vi "setSerializedData.vi"(0 "reference":refnum<class "PackageNode.lvclass">, 1 "parent":refnum<class "AbstractNode.lvclass">, 2 "children":refnum<class "AbstractNode.lvclass">[](array[class]), 3 "xmlOut":string, 5 "error in (no error)":errorcluster) -> (14 "reference out":refnum<class "PackageNode.lvclass">, 19 "error out":errorcluster)   [LabVIEW 2014, in "PackageNode.lvclass"]
doc: "setSerializedData"
uses:
  <resource>/Framework/Providers/Open_GDS/UML/PackageNode_class/PackageNode.lvclass
  <resource>/Framework/Providers/Open_GDS/UML/AbstractNode_class/AbstractNode.lvclass
  <resource>/Framework/Providers/Open_GDS/UML/General/Rectangle/Rectangle Rectangle2D.ctl
  <resource>/Framework/Providers/Open_GDS/UML/MultiLineString_class/JustificationType.ctl
  <resource>/Framework/Providers/Open_GDS/UML/MultiLineString_class/MultiLineString.lvclass
  <resource>/Framework/Providers/Open_GDS/UML/RectangularNode_class/RectangularNode.lvclass
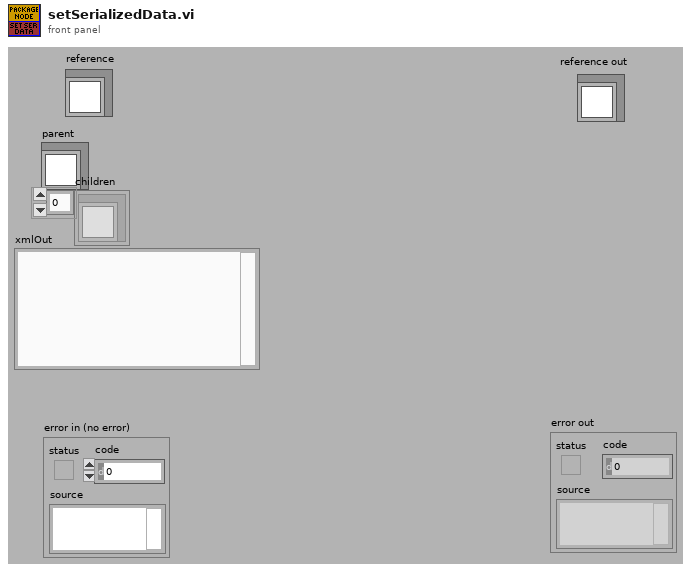
[diagram p1: front panel]
types:
  T1 = typedef "Rectangle Rectangle2D.ctl" = cluster{"x":dbl, "y":dbl, "width":dbl, "height":dbl}
  T2 = cluster{"Base class":cluster{"Base class":cluster{"parent":refnum<k1>, "children":refnum<k1>[], "Hidden":bool}, "bounds":T1}, "name":string, "contents":refnum<k1>, "DEFAULT_TOP_WIDTH":i32, "DEFAULT_TOP_HEIGHT":i32, "DEFAULT_WIDTH":i32, "DEFAULT_HEIGHT":i32, "NAME_GAP":i32, "XGAP":i32, "YGAP":i32, "Collapsed":bool, "Note color":u32, "Justification":u16}
  T3 = cluster{"Base class":cluster{"Base class":cluster{"parent":refnum<k1>, "children":refnum<k1>[], "Hidden":bool}, "bounds":T1}, "name":string, "contents":refnum<k1>, "DEFAULT_TOP_WIDTH":i32, "DEFAULT_TOP_HEIGHT":i32, "DEFAULT_WIDTH":i32, "DEFAULT_HEIGHT":i32, "NAME_GAP":i32, "XGAP":i32, "YGAP":i32, "Collapsed":bool}
  T4 = typedef "MultiLineString.lvclass/JustificationType.ctl" = enum16{"LEFT", "CENTER", "RIGHT"}
  T5 = cluster{"Attributes":cluster{"Base class":cluster{"Base class":cluster{"parent":refnum<k1>, "children":refnum<k1>[], "Hidden":bool}, "bounds":T1}, "name":string, "contents":refnum<k1>, "DEFAULT_TOP_WIDTH":i32, "DEFAULT_TOP_HEIGHT":i32, "DEFAULT_WIDTH":i32, "DEFAULT_HEIGHT":i32, "NAME_GAP":i32, "XGAP":i32, "YGAP":i32, "Collapsed":bool, "Note color":u32, "Justification":u16}, string}
  T6 = typedef "RectangularNode.lvclass/ObjectAttributes.ctl" = cluster{"bounds":T1}
  T7 = typedef "AbstractNode.lvclass/ObjectAttributes.ctl" = cluster{"parent":refnum<class "AbstractNode.lvclass">, "children":refnum<class "AbstractNode.lvclass">[], "Hidden":bool}
  T8 = typedef "PackageNode.lvclass/ObjectAttributes.ctl" = cluster{"name":string, "contents":refnum<class "MultiLineString.lvclass">, "DEFAULT_TOP_WIDTH":i32, "DEFAULT_TOP_HEIGHT":i32, "DEFAULT_WIDTH":i32, "DEFAULT_HEIGHT":i32, "NAME_GAP":i32, "XGAP":i32, "YGAP":i32, "Collapsed":bool, "Note color":u32, "Justification":u16}
  T9 = cluster{"Attributes":cluster{"Base class":cluster{"Base class":cluster{"parent":refnum<k1>, "children":refnum<k1>[], "Hidden":bool}, "bounds":T1}, "name":string, "contents":refnum<k1>, "DEFAULT_TOP_WIDTH":i32, "DEFAULT_TOP_HEIGHT":i32, "DEFAULT_WIDTH":i32, "DEFAULT_HEIGHT":i32, "NAME_GAP":i32, "XGAP":i32, "YGAP":i32, "Collapsed":bool}, string}
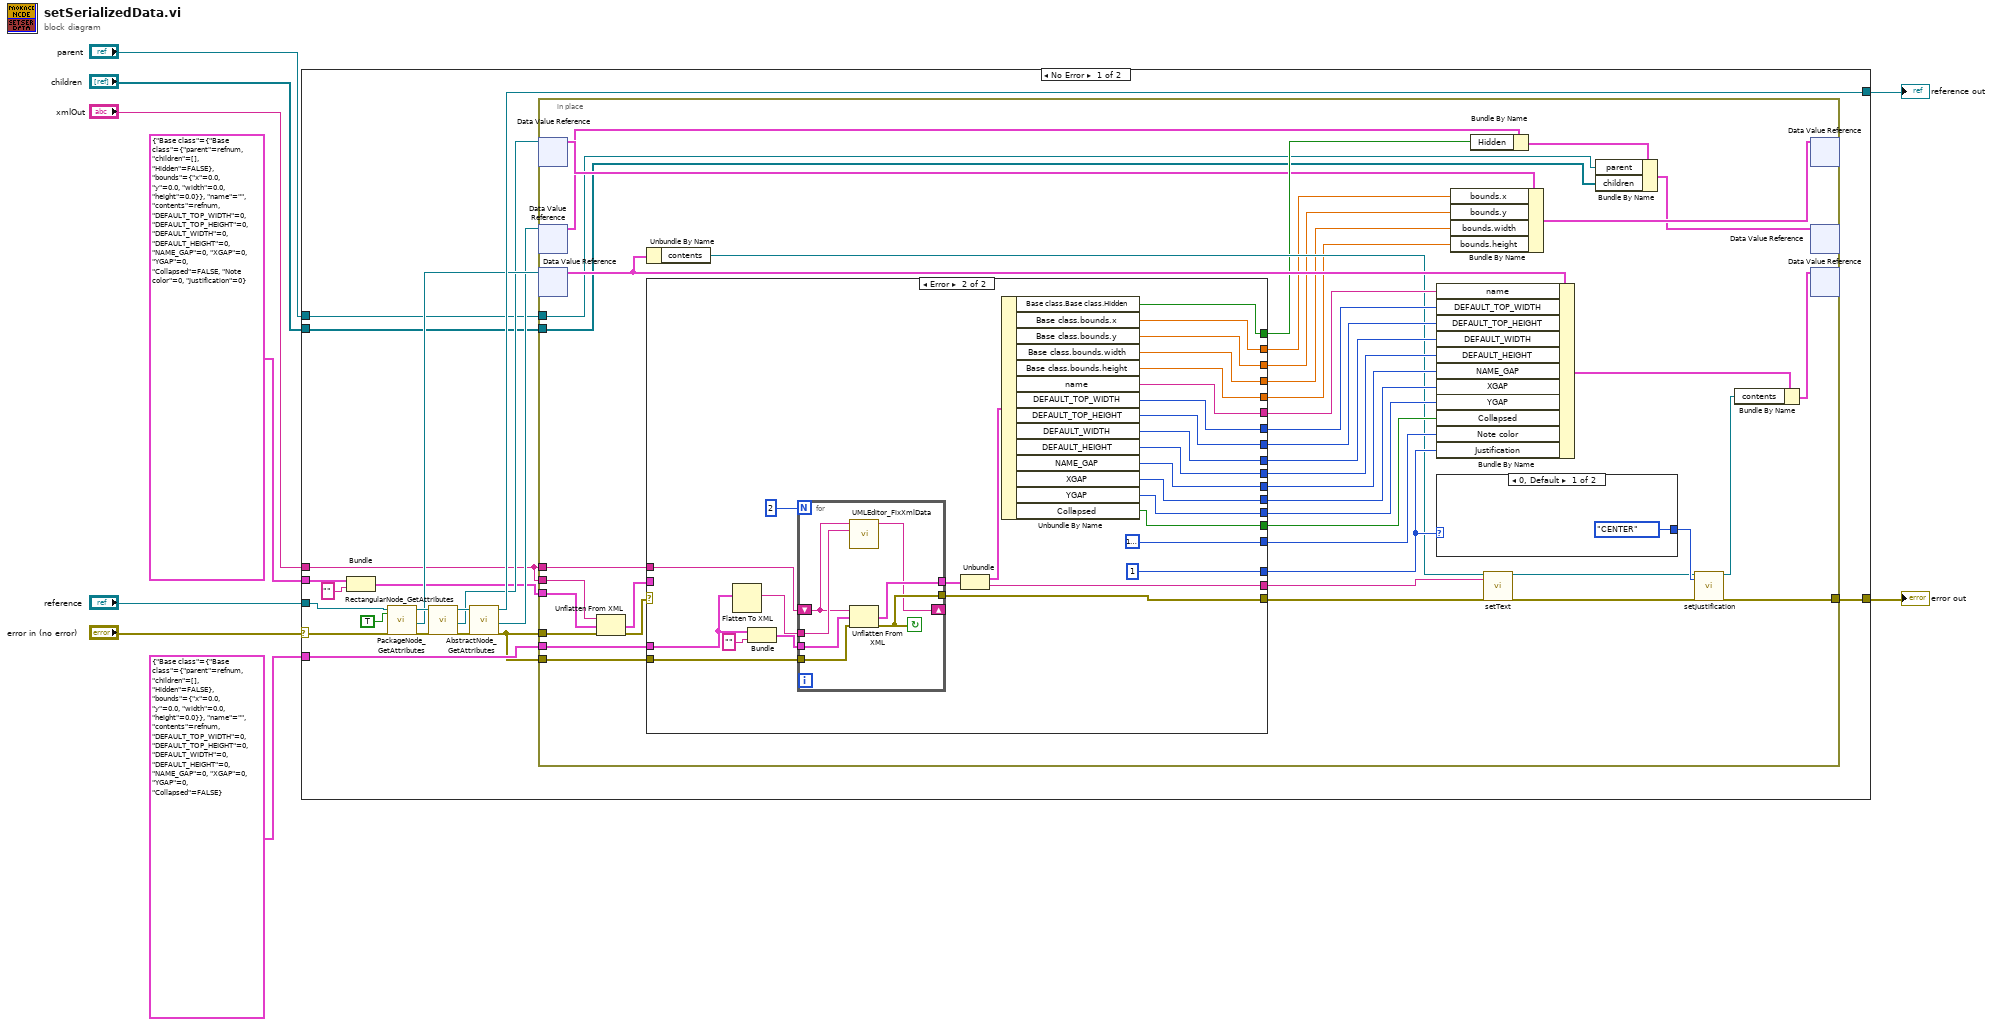
[diagram p0: block diagram]
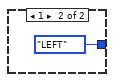
[diagram p2: hidden frame]
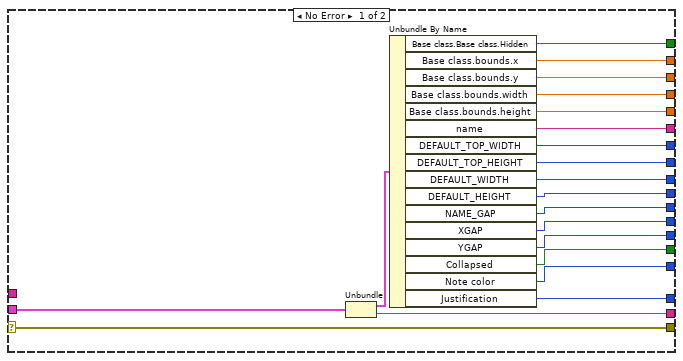
[diagram p3: hidden frame]
diagram:
  n1 = case shown="No Error" "error in (no error)" {
    selector: "error in (no error)" -> [w28 w128]
    tunnel: "reference" -> [w29 w129]
    tunnel: [w27 w128] -> w7
    tunnel: [w26 w129] -> w6
    tunnel: "xmlOut" -> [w12 _]
    tunnel: "parent" -> [w11 _]
    tunnel: "children" -> [w10 _]
    tunnel: T2 {"Base class"={"Base class"={"parent"=refnum, "children"=[], "Hidden"=FALSE}, "bounds"={"x"=0.0, "y"=0.0, "width"=0.0, "height"=0.0}}, "name"="", "contents"=refnum, "DEFAULT_TOP_WIDTH"=0, "DEFAULT_TOP_HEIGHT"=0, "DEFAULT_WIDTH"=0, "DEFAULT_HEIGHT"=0, "NAME_GAP"=0, "XGAP"=0, "YGAP"=0, "Collapsed"=FALSE, "Note color"=0, "Justification"=0} ("Attributes") -> [w24 _]
    tunnel: T3 {"Base class"={"Base class"={"parent"=refnum, "children"=[], "Hidden"=FALSE}, "bounds"={"x"=0.0, "y"=0.0, "width"=0.0, "height"=0.0}}, "name"="", "contents"=refnum, "DEFAULT_TOP_WIDTH"=0, "DEFAULT_TOP_HEIGHT"=0, "DEFAULT_WIDTH"=0, "DEFAULT_HEIGHT"=0, "NAME_GAP"=0, "XGAP"=0, "YGAP"=0, "Collapsed"=FALSE} ("Attributes") -> [w15 _]
    frame No Error {
      n2 = Bundle("Attributes"=w24, "") -> (w13:T5)  [unwired: 1 out]
      n3 = call <resource>:"PackageNode_GetAttributes.vi"("reference in"=w29, "OnlyGetDvrReference(False)"=TRUE, "error in (no error)"=w28) -> ("reference out"=w22:refnum<class "PackageNode.lvclass">, "DataRef"=w18:refnum<data-value>, "error out"=w21:errorcluster)  [unwired: 13 in, 1 out]
      n4 = call <resource>:"RectangularNode_GetAttributes.vi"("reference in"=w22, "error in (no error)"=w21) -> ("reference out"=w20:refnum<class "PackageNode.lvclass">, "DataRef"=w17:refnum<data-value>, "error out"=w19:errorcluster)  [unwired: 14 in, 1 out]
      n5 = call <resource>:"AbstractNode_GetAttributes.vi"("reference in"=w20, "error in (no error)"=w19) -> ("reference out"=w26:refnum<class "PackageNode.lvclass">, "DataRef"=w16:refnum<data-value>, "error out"=w14:errorcluster)  [unwired: 14 in, 1 out]
      n6 = in-place {
        in-place-border: w14 -> [w53]
        in-place-border: w15 -> [w52]
        in-place-border: w12 -> [w51]
        in-place-border: [w40] -> w27
        in-place-border: w14 -> [w39]
        in-place-border: w13 -> [w38]
        in-place-border: w12 -> [w37]
        in-place-border: w11 -> [w33]
        in-place-border: w10 -> [w32]
        n7 = in-place-dvr #1(w17) -> (w36:T6)  [unwired: 1 out]
        n8 = in-place-dvr #2(w16) -> (w35:T7)  [unwired: 1 out]
        n9 = in-place-dvr #3(w18) -> (w71:T8)  [unwired: 1 out]
        n10 = Unflatten From XML(xml string=w37, type=w38, error in (no error)=w39) -> (value=w54:T5, error out=w55:errorcluster)
        n11 = Unbundle By Name(w71) -> ("contents"=w58:refnum<class "MultiLineString.lvclass">)
        n12 = case shown="Error" w55 {
          selector: w55 -> [w76 _]
          tunnel: w54 -> [w93 _]
          tunnel: [w92 w119] -> w50
          tunnel: [w90 w105] -> w49
          tunnel: [w89 w117] -> w48
          tunnel: [w88 w106] -> w47
          tunnel: [w87 w107] -> w46
          tunnel: [w86 w116] -> w70
          tunnel: [w85 w108] -> w69
          tunnel: [w84 w115] -> w68
          tunnel: [w83 w109] -> w67
          tunnel: [w82 w114] -> w66
          tunnel: [w81 w110] -> w65
          tunnel: [w80 w111] -> w64
          tunnel: [w79 w112] -> w63
          tunnel: [w78 w113] -> w62
          tunnel: [w77 w118] -> w45
          tunnel: [w76 w98] -> w44
          tunnel: w53 -> [_ w99]
          tunnel: w52 -> [_ w101]
          tunnel: w51 -> [_ w95]
          tunnel: [w75 u32 16777216] -> w61
          tunnel: [w74 u16 1 ("Justification")] -> w60
          frame No Error {
            n13 = Unbundle(w93) -> ("Attributes"=w91:T2, w92:string)
            n14 = Unbundle By Name(w91) -> ("Base class.Base class.Hidden"=w77:bool, "Base class.bounds.x"=w90:dbl, "Base class.bounds.y"=w89:dbl, "Base class.bounds.width"=w88:dbl, "Base class.bounds.height"=w87:dbl, "name"=w86:string, "DEFAULT_TOP_WIDTH"=w85:i32, "DEFAULT_TOP_HEIGHT"=w84:i32, "DEFAULT_WIDTH"=w83:i32, "DEFAULT_HEIGHT"=w82:i32, "NAME_GAP"=w81:i32, "XGAP"=w80:i32, "YGAP"=w79:i32, "Collapsed"=w78:bool, "Note color"=w75:u32, "Justification"=w74:u16)
          }
          frame Error {
            n15 = Flatten To XML(anything=w101) -> (xml string=w94:string)
            n16 = Bundle("Attributes"=w101, "") -> (w97:T9)  [unwired: 1 out]
            n17 = for {
              N: 2 -> [_]
              tunnel: w99 -> [w127]
              tunnel: [w123] -> w98
              tunnel: [w126] -> w96
              tunnel: w94 -> [w125]
              tunnel: w97 -> [w124]
              shift-right: [w122] -> _
              shift-left: w95 -> [w121]
              stop <- w123 continue-if-true
              n18 = call <resource>:"UMLEditor_FixXmlData.vi"("XmlTemplateIn"=w125, "xmlIn"=w121) -> ("XML OUt"=w122:string)  [unwired: 9 in]
              n19 = Unflatten From XML(xml string=w121, type=w124, error in (no error)=w127) -> (value=w126:T9, error out=w123:errorcluster)
            }
            n20 = Unbundle(w96) -> ("Attributes"=w104:T3, w119:string)
            n21 = Unbundle By Name(w104) -> ("Base class.Base class.Hidden"=w118:bool, "Base class.bounds.x"=w105:dbl, "Base class.bounds.y"=w117:dbl, "Base class.bounds.width"=w106:dbl, "Base class.bounds.height"=w107:dbl, "name"=w116:string, "DEFAULT_TOP_WIDTH"=w108:i32, "DEFAULT_TOP_HEIGHT"=w115:i32, "DEFAULT_WIDTH"=w109:i32, "DEFAULT_HEIGHT"=w114:i32, "NAME_GAP"=w110:i32, "XGAP"=w111:i32, "YGAP"=w112:i32, "Collapsed"=w113:bool)
          }
        }
        n22 = Bundle By Name(cluster=w71, "name"=w70, "DEFAULT_TOP_WIDTH"=w69, "DEFAULT_TOP_HEIGHT"=w68, "DEFAULT_WIDTH"=w67, "DEFAULT_HEIGHT"=w66, "NAME_GAP"=w65, "XGAP"=w64, "YGAP"=w63, "Collapsed"=w62, "Note color"=w61, "Justification"=w60) -> (w59:T8)
        n23 = case shown="0, Default" w60 {
          tunnel: [JustificationType."CENTER" ("justification") JustificationType."LEFT" ("justification")] -> w43
          frame 0, Default {
          }
          frame 1 {
          }
        }
        n24 = Bundle By Name(cluster=w36, "bounds.x"=w49, "bounds.y"=w48, "bounds.width"=w47, "bounds.height"=w46) -> (w31:T6)
        n25 = Bundle By Name(cluster=w35, "Hidden"=w45) -> (w34:T7)
        n26 = call-dynamic "setText.vi"("reference"=w58, "text"=w50, "error in (no error)"=w44) -> ("reference out"=w42:refnum<class "MultiLineString.lvclass">, "error out"=w41:errorcluster)  [unwired: 15 out]
        n27 = Bundle By Name(cluster=w34, "parent"=w33, "children"=w32) -> (w30:T7)
        n28 = call <resource>:"setJustification.vi"("reference"=w42, "justification"=w43, "error in (no error)"=w41) -> ("reference out"=w57:refnum<class "MultiLineString.lvclass">, "error out"=w40:errorcluster)  [unwired: 15 out]
        n29 = Bundle By Name(cluster=w59, "contents"=w57) -> (w56:T8)
        n30 = in-place-dvr #1(w31) -> ()  [unwired: 2 out]
        n31 = in-place-dvr #2(w30) -> ()  [unwired: 2 out]
        n32 = in-place-dvr #3(w56) -> ()  [unwired: 2 out]
      }
    }
    frame Error {
    }
  }
  "reference out" <- w6
  "error out" <- w7
